vi "SParam Test Configuration.vi"(8 "error in":errorcluster, 10 "Test Configuration":T2={"Action"=enum."Measure", "Power Level (dBm)"=0.0, "External Gain (dB)"=0.0, "Frequency Sweep"={"Start Frequency (Hz)"=0.0, "Stop Frequency (Hz)"=0.0, "Step Size (Hz)"=0.0}, "Type of Stimulus"=enum."CW", "Pulse Width (s)"=0.0, "PRI (s)"=10.0, "IF Bandwidth (Hz)"=10.0, "Average Mode"=enum."Per Sweep", "Number of Averages"=0, "SnP File Path"=path "", "Calibration File Path"=path ""} {"Frequency Sweep"."Step Size (Hz)" format="%#_6p"; "Frequency Sweep"."Stop Frequency (Hz)" format="%.3p"; "Frequency Sweep"."Start Frequency (Hz)" format="%.3p"}, 11 "S-Par Reference In":T1) -> (0 "error out":errorcluster, 3 "S-Par Reference Out":T1)   [LabVIEW 2023]
uses:
  Controls/Test Config - SParam_VST.ctl
  <vilib>/niSPML/Typedefs/Session Handle.ctl
  <vilib>/niSPML/S-Par Reference.lvclass
  <vilib>/niSPML/S-Parameter Measurements.lvlib
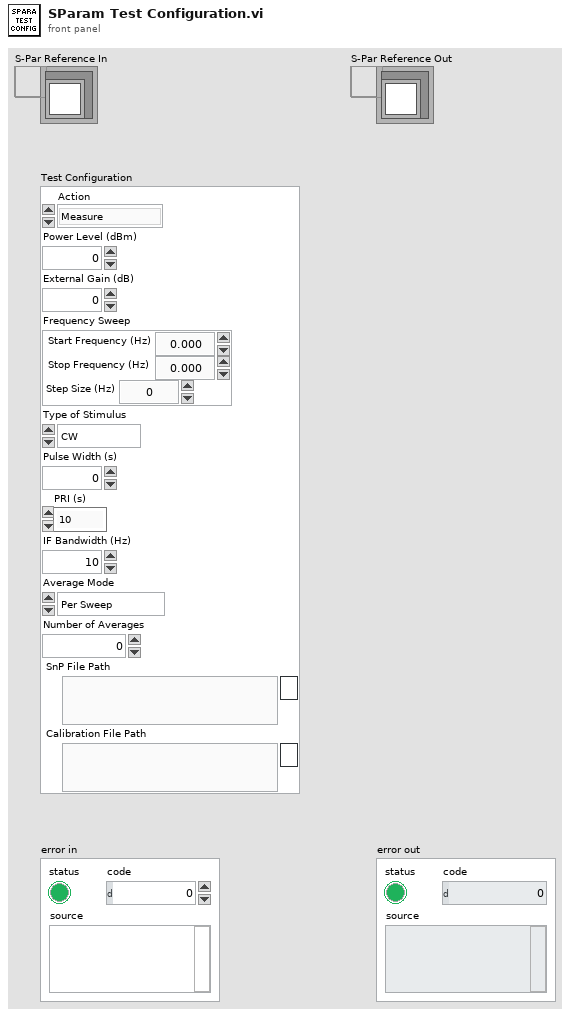
[diagram p1: front panel]
types:
  T1 = typedef "S-Parameter Measurements.lvlib/S-Par Reference.lvclass/Session Handle.ctl" = refnum<data-value>
  T2 = typedef "Test Config - SParam_VST.ctl" = cluster{"Action":enum32{"Calibrate", "Measure"}, "Power Level (dBm)":dbl, "External Gain (dB)":dbl, "Frequency Sweep":cluster{"Start Frequency (Hz)":dbl, "Stop Frequency (Hz)":dbl, "Step Size (Hz)":dbl}, "Type of Stimulus":enum16{"CW", "Pulsed CW"}, "Pulse Width (s)":dbl, "PRI (s)":dbl, "IF Bandwidth (Hz)":dbl, "Average Mode":enum16{"Per Sweep", "Per Point"}, "Number of Averages":i32, "SnP File Path":path, "Calibration File Path":path}
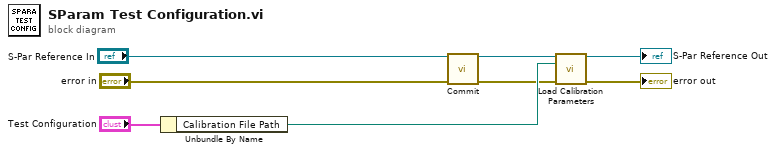
[diagram p0: block diagram]
diagram:
  n1 = Unbundle By Name("Test Configuration") -> ("Calibration File Path"=w5:path)
  n2 = call <vilib>:"Commit.vi"("S-Par Reference In"="S-Par Reference In", "error in"="error in") -> ("S-Par Reference Out"=w2:T1, "error out"=w1:errorcluster)  [unwired: 12 in]
  n3 = call <vilib>:"Load Calibration Parameters.vi"("S-Par Reference In"=w2, "Calibration Parameters File Path"=w5, "error in"=w1) -> ("S-Par Reference Out"=→"S-Par Reference Out":T1, "error out"=→"error out":errorcluster)  [unwired: 11 in]
